vi "#81701_MAV_MSG_MORTAR_CMD_DROP_ENCODE.vi"(10 "packet_sequence_in":u8, 11 "MORTAR_CMD_DROP":T1={"mortar_stage"={"MORTAR_STAGE_1"=TRUE, "MORTAR_STAGE_2"=TRUE, "MORTAR_STAGE_3"=TRUE, "MORTAR_STAGE_4"=TRUE, "MORTAR_STAGE_5"=TRUE, "MORTAR_STAGE_6"=TRUE}, "target_system"=1, "target_component"=50, "self"={"system_id"=1, "component_id"=50}}) -> (2 "packet_sequence_out":u8, 3 "mavlink_buffer_out":u8[](array[numeric]))   [LabVIEW 2023]
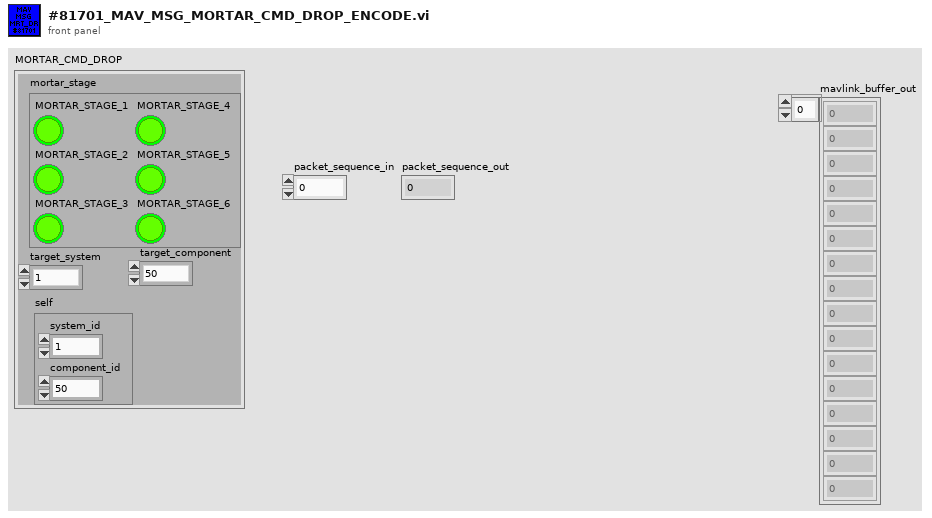
[diagram p1: front panel]
types:
  T1 = cluster{"mortar_stage":cluster{"MORTAR_STAGE_1":bool, "MORTAR_STAGE_2":bool, "MORTAR_STAGE_3":bool, "MORTAR_STAGE_4":bool, "MORTAR_STAGE_5":bool, "MORTAR_STAGE_6":bool}, "target_system":u8, "target_component":u8, "self":cluster{"system_id":u8, "component_id":u8}}
  T2 = cluster{"MORTAR_STAGE_1":bool, "MORTAR_STAGE_2":bool, "MORTAR_STAGE_3":bool, "MORTAR_STAGE_4":bool, "MORTAR_STAGE_5":bool, "MORTAR_STAGE_6":bool}
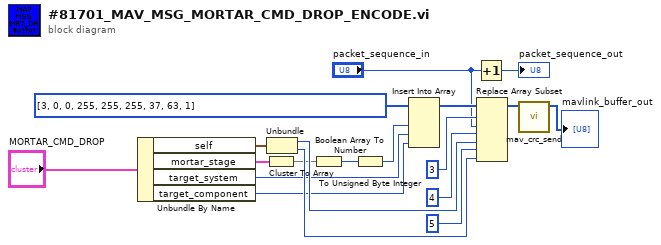
[diagram p0: block diagram]
diagram:
  n1 = Unbundle By Name("MORTAR_CMD_DROP") -> ("self"=w17:cluster{"system_id":u8, "component_id":u8}, "mortar_stage"=w4:T2, "target_system"=w6:u8, "target_component"=w5:u8)
  n2 = Cluster To Array(cluster=w4) -> (array=w3:bool[])
  n3 = Unbundle(w17) -> ("system_id"=w10:u8, "component_id"=w9:u8)
  n4 = Boolean Array To Number(Boolean array=w3) -> (number=w2:u32)
  n5 = To Unsigned Byte Integer(number=w2) -> (unsigned 8bit integer=w1:u8)
  n6 = Insert Into Array(array=u8[] [3, 0, 0, 255, 255, 255, 37, 63, 1], new element #1=w1, new element #2=w6, new element #3=w5) -> (w15:u8[])  [unwired: 1 in]
  n7 = Increment(x="packet_sequence_in") -> (x+1=→"packet_sequence_out":u8)
  n8 = Replace Array Subset(array=w15, new element #1="packet_sequence_in", index #1=3 ("index"), new element #2=w10, index #2=4 ("index"), new element #3=w9, index #3=5 ("index")) -> (w8:u8[])
  n9 = call "mav_crc_send.vi"("Byte In"=w8) -> ("Output Byte"=→"mavlink_buffer_out":u8[])  [unwired: 10 in]
